vi "PF200Test.vi"() -> ()   [LabVIEW 2020]
uses:
  <vilib>/DAQmx/read.llb/DAQmx Read (Analog DBL 1Chan 1Samp).vi
  <vilib>/DAQmx/write.llb/DAQmx Write.vi
  <vilib>/DAQmx/write.llb/DAQmx Write (Digital 1D Bool NChan 1Samp 1Line).vi
panel:
  out "Numeric 11":dbl
  in  "Boolean":bool
  out "Numeric 10":dbl
  out "Numeric 9":dbl
  out "Numeric 8":dbl
  out "Numeric 7":dbl
  out "Numeric 6":dbl
  out "Numeric 5":dbl
  in  "Numeric 4":dbl
  in  "Numeric 3":dbl
  out "Numeric 2":dbl
  out "Numeric":dbl
  in  "stop (F)":bool
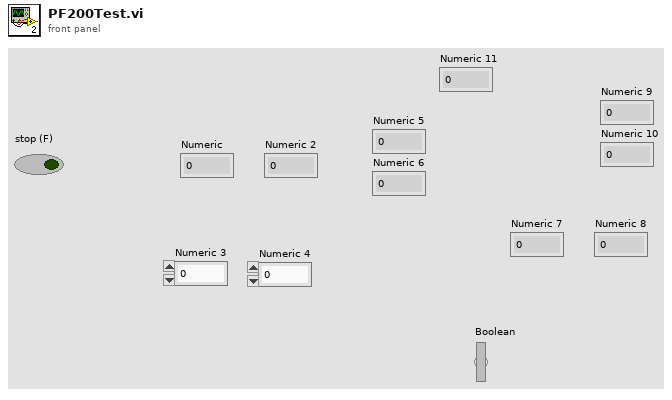
[diagram p1: front panel]
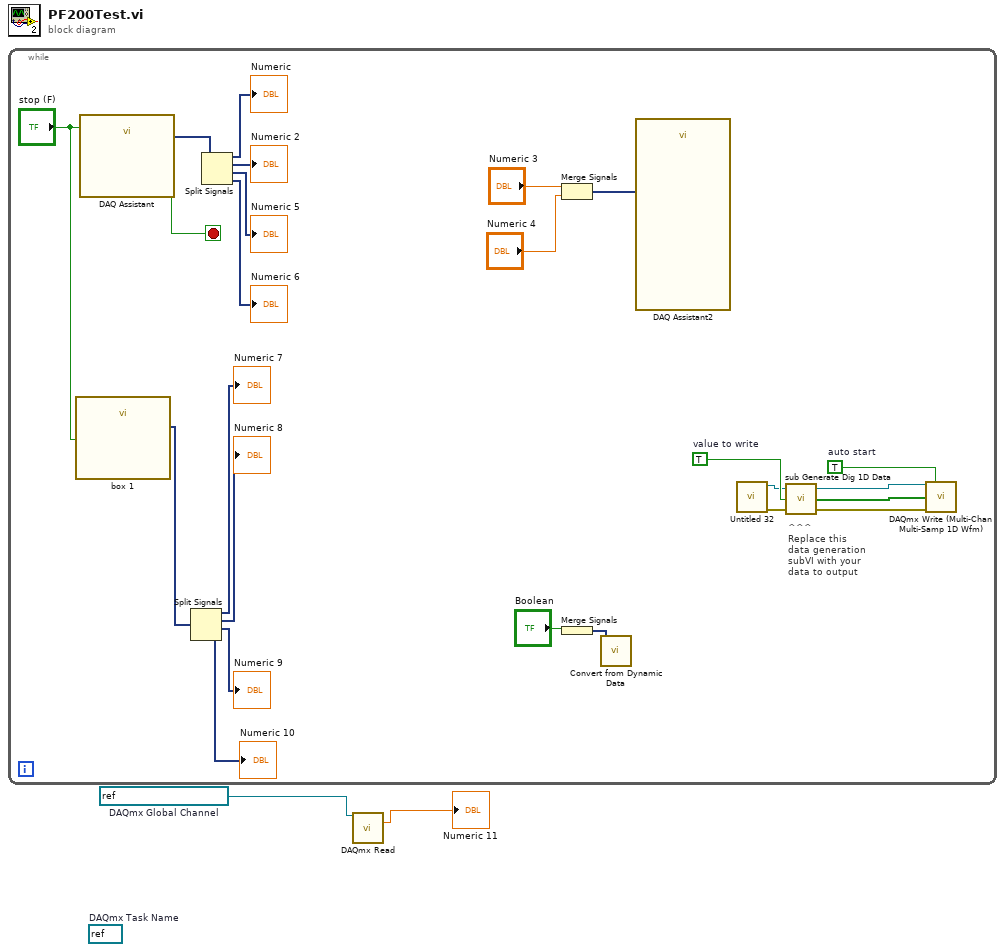
[diagram p0: block diagram]
diagram:
  w2 = refnum<k21> "MyVoltageChannel"  # DAQmx Global Channel
  (unwired) refnum<k21> refnum  # DAQmx Task Name
  n1 = while {
    stop <- w27 stop-if-true
    w8 = TRUE  # value to write
    w9 = TRUE  # auto start
    # "^^^\nReplace this\ndata generation\nsubVI with your\ndata to output"
    n2 = call "box 1"("stop (T)"="stop (F)") -> ("data"=w14:dynamicdata)  [unwired: 16 in, 2 out]
    n3 = call "DAQ Assistant"("stop (F)"="stop (F)") -> ("data"=w26:dynamicdata, "stopped"=w27:bool)  [unwired: 15 in, 2 out]
    n4 = Split Signals(w14) -> (→"Numeric 7":dynamicdata, →"Numeric 8":dynamicdata, →"Numeric 9":dynamicdata, →"Numeric 10":dynamicdata)  [unwired: 4 in]
    n5 = Split Signals(w26) -> (→"Numeric":dynamicdata, →"Numeric 2":dynamicdata, →"Numeric 5":dynamicdata, →"Numeric 6":dynamicdata)  [unwired: 4 in]
    n6 = Merge Signals("Numeric 3", "Numeric 4") -> (w21:dynamicdata)
    n7 = Merge Signals("Boolean") -> (w11:dynamicdata)
    n8 = call "Convert from Dynamic Data"("Dynamic Data Type"=w11) -> ("Array"=w10:bool[])  [unwired: 3 in]
    n9 = call "DAQ Assistant2"("data"=w21) -> ()  [unwired: 17 in, 2 out]
    n10 = call "Untitled 32.vi"() -> ("error out"=w3:errorcluster, "task out"=w4:refnum<k21>)  [unwired: 10 in]
    n11 = call <vilib>:"sub Generate Dig 1D Data.vi"("error in"=w3, "initial value"=w8, "task in"=w4) -> ("error out"=w7:errorcluster, "Data"=w6:bool[], "task out"=w5:refnum<k21>)
    n12 = call-poly "DAQmx Write (Multi-Chan Multi-Samp 1D Wfm).vi"("task/channels in"=w5, "auto start"=w9, "data"=w6, "error in"=w7) -> ()  [unwired: 9 in, 3 out]
  }
  n13 = call-poly <vilib>:"DAQmx Read.vi"("task/channels in"=w2) -> ("data"=→"Numeric 11":dbl)  [unwired: 12 in, 2 out]
